vi "Generate command.vi"(1 "Action":T1, 7 "n(0)":i32, 9 "d(0.0)":dbl, 11 "error IO":errorcluster) -> (8 "Command string":string, 10 "Reply expected":bool, 15 "error out":errorcluster)   [LabVIEW 2011]
uses:
  PCP Commands.ctl
  <vilib>/Utility/VariantDataType/VariantType.lvlib
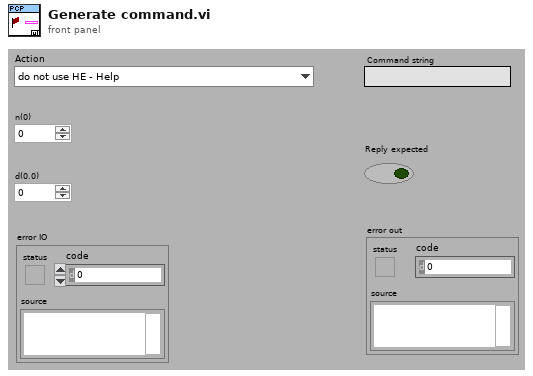
[diagram p1: front panel]
types:
  T1 = typedef "PCP Commands.ctl" = enum16{"do not use HE - Help", "RDd - Most used inputs", "RA - All analog inputs", "RE n Reset DO n", "SE n Set DO n", "RP - Get digital inputs", "VA d Set AO A  Motor Volt", "VB d Set AO B  Cable Resistance", "VEr - Get Version", "DYp - Depth counter", "DR - Reset Depth Counter", "DS n Set Depth options(0-3)", "do not use ME - Manual mode enabled", "MD - Manual mode disabled", "ID - Get ID(2001)", "TS - Get Timestamp", "TO d(s)  Set timeout", "do not use LO n Start Loop Mode(1,2)", "AL n RD&LO variation", "ST - Stop Loop Mode"}
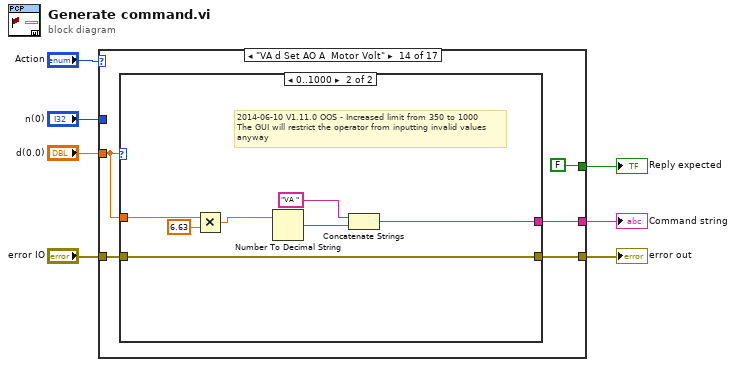
[diagram p0: block diagram]
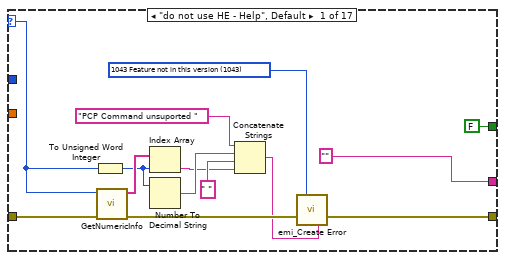
[diagram p2: hidden frame]
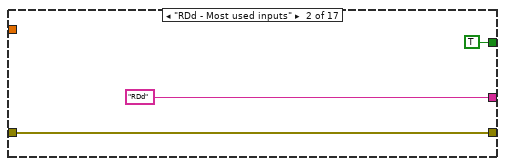
[diagram p3: hidden frame]
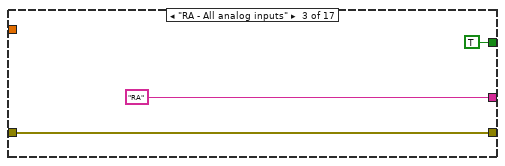
[diagram p4: hidden frame]
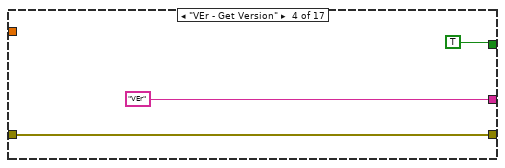
[diagram p5: hidden frame]
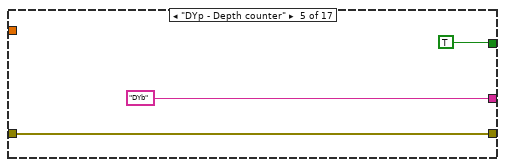
[diagram p6: hidden frame]
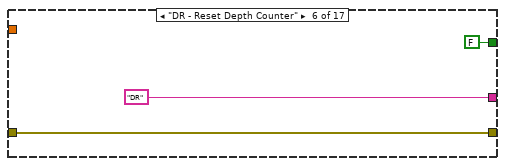
[diagram p7: hidden frame]
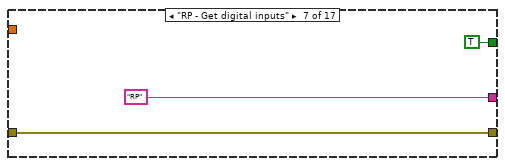
[diagram p8: hidden frame]
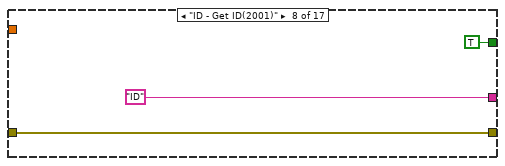
[diagram p9: hidden frame]
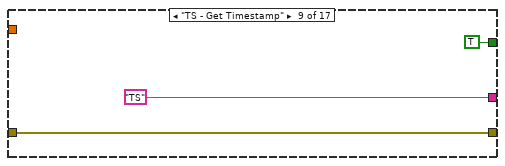
[diagram p10: hidden frame]
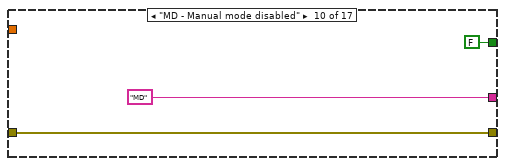
[diagram p11: hidden frame]
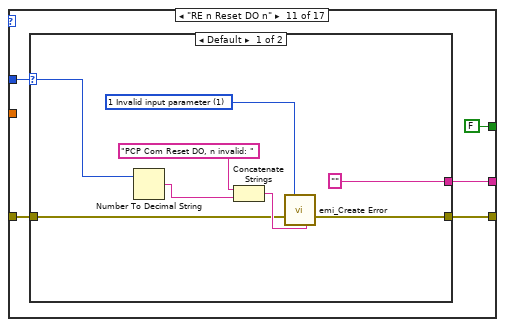
[diagram p12: hidden frame]
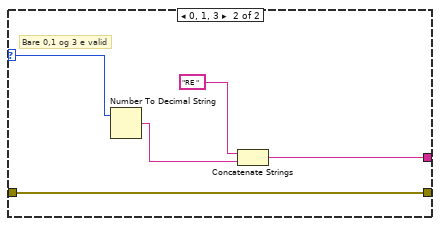
[diagram p13: hidden frame]
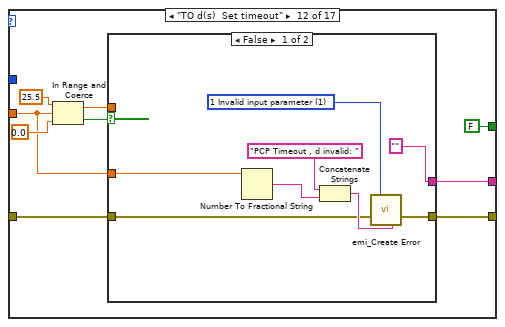
[diagram p14: hidden frame]
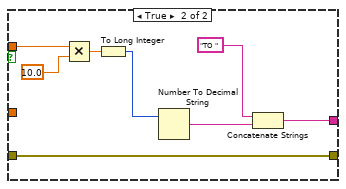
[diagram p15: hidden frame]
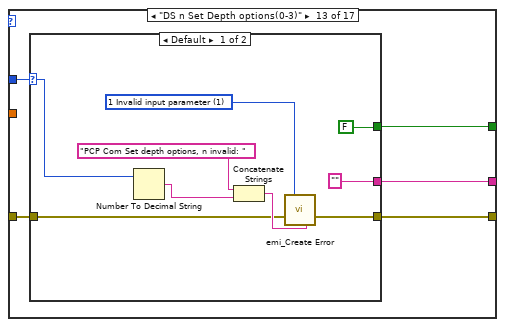
[diagram p16: hidden frame]
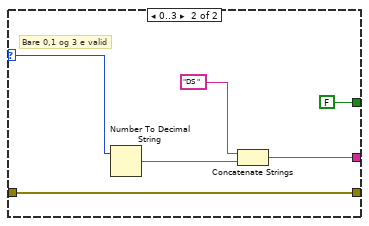
[diagram p17: hidden frame]
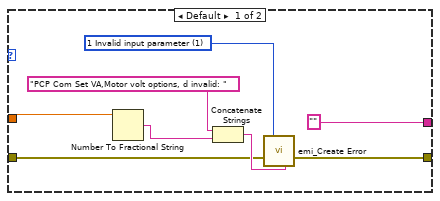
[diagram p18: hidden frame]
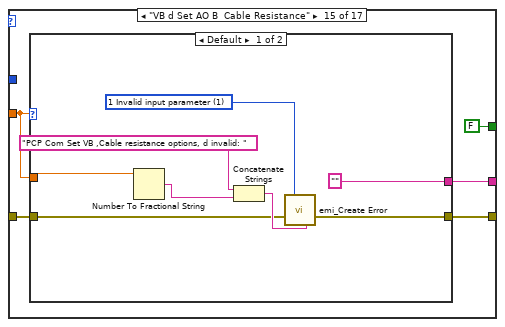
[diagram p19: hidden frame]
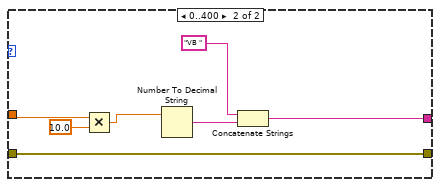
[diagram p20: hidden frame]
diagram:
  n1 = case shown="\"VA d Set AO A  Motor Volt\"" "Action" {
    selector: "Action" -> [w17 _ _ _ _ _ _ _ _ _ _ _ _ _ _ _ _]
    tunnel: "error IO" -> [w19 w24 w27 w30 w33 w36 w39 w42 w45 w48 w51 w74 w94 w115 w135 w154 w172]
    tunnel: [w21 w24 w27 w30 w33 w36 w39 w42 w45 w48 w50 w73 w93 w114 w134 w153 w171] -> w6
    tunnel: "n(0)" -> [_ _ _ _ _ _ _ _ _ _ w52 _ w95 _ _ w155 w173]
    tunnel: ["" "RDd" "RA" "VEr" "DYb" "DR" "RP" "ID" "TS" "MD" w53 w75 w96 w116 w136 w156 w174] -> w7
    tunnel: "d(0.0)" -> [_ _ _ _ _ _ _ _ _ _ _ w67 _ w113 w133 _ _]
    tunnel: [FALSE ("Reply expected") TRUE ("Reply expected") TRUE ("Reply expected") TRUE ("Reply expected") TRUE ("Reply expected") FALSE ("Reply expected") TRUE ("Reply expected") TRUE ("Reply expected") TRUE ("Reply expected") FALSE ("Reply expected") FALSE ("Reply expected") FALSE ("Reply expected") w92 FALSE ("Reply expected") FALSE ("Reply expected") FALSE ("Reply expected") FALSE ("Reply expected")] -> w1
    frame "do not use HE - Help", Default {
      w20 = 1043 items=["0 No Error"=0, "7 File not Found"=7, "35 Generic Pring Error"=35, "37 Device not Found"=37, "39 Device Unit Error"=39, "40 Could fot Open Device"=40, "42 Generic Error"=42, "52 Unknown Message"=52, "98 Bad File type"=98, "99 Bad File Version"=99, "100 Bad Data in File"=100, "1018 Unspecefied Error"=1018, "1041 Incorrect Password"=1041, "1043 Feature not in this version"=1043] ("Error Code")
      n2 = To Unsigned Word Integer(number=w17) -> (unsigned 16bit integer=w15:u16)
      n3 = call <vilib>:"GetNumericInfo.vi"("error in (no error)"=w19, "Variant"=w17) -> ("error out"=w18:errorcluster, "EnumNames"=w16:string[])  [unwired: 6 in, 2 out]
      n4 = Index Array(array=w16, index=w15) -> (element=w11:string)
      n5 = Number To Decimal String(number=w15) -> (decimal integer string=w13:string)  [unwired: 1 in]
      n6 = Concatenate Strings("PCP Command unsuported " ("string"), w13, " " ("string"), w11) -> (w10:string)
      n7 = call "emi_Create Error.vi"("Error Code"=w20, "error in (no error)"=w18, "Append String(\"\")"=w10) -> ("error out"=w21:errorcluster)  [unwired: 12 in]
    }
    frame "RDd - Most used inputs" {
    }
    frame "RA - All analog inputs" {
    }
    frame "VEr - Get Version" {
    }
    frame "DYp - Depth counter" {
    }
    frame "DR - Reset Depth Counter" {
    }
    frame "RP - Get digital inputs" {
    }
    frame "ID - Get ID(2001)" {
    }
    frame "TS - Get Timestamp" {
    }
    frame "MD - Manual mode disabled" {
    }
    frame "RE n Reset DO n" {
      n8 = case shown="Default" w52 {
        selector: w52 -> [w56 w64]
        tunnel: ["" w65] -> w53
        tunnel: w51 -> [w54 w62]
        tunnel: [w55 w62] -> w50
        frame Default {
          w60 = 1 items=["0 No Error"=0, "1 Invalid input parameter"=1, "6 Generic file IO "=6, "7 File not Found"=7, "35 Generic Pring Error"=35, "37 Device not Found"=37, "39 Device Unit Error"=39, "40 Could fot Open Device"=40, "42 Generic Error"=42, "52 Unknown Message"=52, "98 Bad File type"=98, "99 Bad File Version"=99, "100 Bad Data in File"=100, "1018 Unspecefied Error"=1018, "1041 Incorrect Password"=1041, "1043 Feature not in this version"=1043] ("Error Code")
          n9 = Number To Decimal String(number=w56) -> (decimal integer string=w57:string)  [unwired: 1 in]
          n10 = Concatenate Strings("PCP Com Reset DO, n invalid: " ("string"), w57) -> (w59:string)
          n11 = call "emi_Create Error.vi"("Error Code"=w60, "error in (no error)"=w54, "Append String(\"\")"=w59) -> ("error out"=w55:errorcluster)  [unwired: 12 in]
        }
        frame 0, 1, 3 {
          # "Bare 0,1 og 3 e valid"
          n12 = Number To Decimal String(number=w64) -> (decimal integer string=w63:string)  [unwired: 1 in]
          n13 = Concatenate Strings("RE ", w63) -> (w65:string)
        }
      }
    }
    frame "TO d(s)  Set timeout" {
      n14 = In Range and Coerce(upper limit=25.5, x=w67, lower limit=0.0) -> (coerced(x)=w69:dbl, In Range?=w68:bool)
      n15 = case shown="False" w68 {
        tunnel: ["" w90] -> w75
        tunnel: w74 -> [w76 w89]
        tunnel: [w77 w89] -> w73
        tunnel: w69 -> [_ w88]
        tunnel: w67 -> [w78 _]
        frame False {
          w82 = 1 items=["0 No Error"=0, "1 Invalid input parameter"=1, "6 Generic file IO "=6, "7 File not Found"=7, "35 Generic Pring Error"=35, "37 Device not Found"=37, "39 Device Unit Error"=39, "40 Could fot Open Device"=40, "42 Generic Error"=42, "52 Unknown Message"=52, "98 Bad File type"=98, "99 Bad File Version"=99, "100 Bad Data in File"=100, "1018 Unspecefied Error"=1018, "1041 Incorrect Password"=1041, "1043 Feature not in this version"=1043] ("Error Code")
          n16 = Number To Fractional String(number=w78) -> (F-format string=w79:string)  [unwired: 3 in]
          n17 = Concatenate Strings("PCP Timeout , d invalid: " ("string"), w79) -> (w81:string)
          n18 = call "emi_Create Error.vi"("Error Code"=w82, "error in (no error)"=w76, "Append String(\"\")"=w81) -> ("error out"=w77:errorcluster)  [unwired: 12 in]
        }
        frame True {
          n19 = Multiply(x=w88, y=10.0) -> (x*y=w85:dbl)
          n20 = To Long Integer(number=w85) -> (32bit integer=w84:i32)
          n21 = Number To Decimal String(number=w84) -> (decimal integer string=w86:string)  [unwired: 1 in]
          n22 = Concatenate Strings("TO ", w86) -> (w90:string)
        }
      }
    }
    frame "DS n Set Depth options(0-3)" {
      n23 = case shown="Default" w95 {
        selector: w95 -> [w100 w109]
        tunnel: ["" w110] -> w96
        tunnel: w94 -> [w97 w107]
        tunnel: [w98 w107] -> w93
        tunnel: [FALSE ("Reply expected") FALSE ("Reply expected")] -> w92
        frame Default {
          w104 = 1 items=["0 No Error"=0, "1 Invalid input parameter"=1, "6 Generic file IO "=6, "7 File not Found"=7, "35 Generic Pring Error"=35, "37 Device not Found"=37, "39 Device Unit Error"=39, "40 Could fot Open Device"=40, "42 Generic Error"=42, "52 Unknown Message"=52, "98 Bad File type"=98, "99 Bad File Version"=99, "100 Bad Data in File"=100, "1018 Unspecefied Error"=1018, "1041 Incorrect Password"=1041, "1043 Feature not in this version"=1043] ("Error Code")
          n24 = Number To Decimal String(number=w100) -> (decimal integer string=w101:string)  [unwired: 1 in]
          n25 = Concatenate Strings("PCP Com Set depth options, n invalid: " ("string"), w101) -> (w103:string)
          n26 = call "emi_Create Error.vi"("Error Code"=w104, "error in (no error)"=w97, "Append String(\"\")"=w103) -> ("error out"=w98:errorcluster)  [unwired: 12 in]
        }
        frame 0..3 {
          # "Bare 0,1 og 3 e valid"
          n27 = Number To Decimal String(number=w109) -> (decimal integer string=w108:string)  [unwired: 1 in]
          n28 = Concatenate Strings("DS ", w108) -> (w110:string)
        }
      }
    }
    frame "VA d Set AO A  Motor Volt" {
      n29 = case shown="0..1000" w113 {
        tunnel: ["" w130] -> w116
        tunnel: w115 -> [w117 w128]
        tunnel: [w118 w128] -> w114
        tunnel: w113 -> [w119 w127]
        frame Default {
          w123 = 1 items=["0 No Error"=0, "1 Invalid input parameter"=1, "6 Generic file IO "=6, "7 File not Found"=7, "35 Generic Pring Error"=35, "37 Device not Found"=37, "39 Device Unit Error"=39, "40 Could fot Open Device"=40, "42 Generic Error"=42, "52 Unknown Message"=52, "98 Bad File type"=98, "99 Bad File Version"=99, "100 Bad Data in File"=100, "1018 Unspecefied Error"=1018, "1041 Incorrect Password"=1041, "1043 Feature not in this version"=1043] ("Error Code")
          n30 = Number To Fractional String(number=w119) -> (F-format string=w120:string)  [unwired: 3 in]
          n31 = Concatenate Strings("PCP Com Set VA,Motor volt options, d invalid: " ("string"), w120) -> (w122:string)
          n32 = call "emi_Create Error.vi"("Error Code"=w123, "error in (no error)"=w117, "Append String(\"\")"=w122) -> ("error out"=w118:errorcluster)  [unwired: 12 in]
        }
        frame 0..1000 {
          # "2014-06-10 V1.11.0 OOS - Increased limit from 350 to 1000\nThe GUI will restrict the operator from inputting invalid values\nanyway"
          n33 = Multiply(x=w127, y=6.63) -> (x*y=w125:dbl)
          n34 = Number To Decimal String(number=w125) -> (decimal integer string=w129:string)  [unwired: 1 in]
          n35 = Concatenate Strings("VA ", w129) -> (w130:string)
        }
      }
    }
    frame "VB d Set AO B  Cable Resistance" {
      n36 = case shown="Default" w133 {
        tunnel: ["" w150] -> w136
        tunnel: w135 -> [w138 w148]
        tunnel: [w137 w148] -> w134
        tunnel: w133 -> [w139 w147]
        frame Default {
          w143 = 1 items=["0 No Error"=0, "1 Invalid input parameter"=1, "6 Generic file IO "=6, "7 File not Found"=7, "35 Generic Pring Error"=35, "37 Device not Found"=37, "39 Device Unit Error"=39, "40 Could fot Open Device"=40, "42 Generic Error"=42, "52 Unknown Message"=52, "98 Bad File type"=98, "99 Bad File Version"=99, "100 Bad Data in File"=100, "1018 Unspecefied Error"=1018, "1041 Incorrect Password"=1041, "1043 Feature not in this version"=1043] ("Error Code")
          n37 = Number To Fractional String(number=w139) -> (F-format string=w140:string)  [unwired: 3 in]
          n38 = Concatenate Strings("PCP Com Set VB ,Cable resistance options, d invalid: " ("string"), w140) -> (w142:string)
          n39 = call "emi_Create Error.vi"("Error Code"=w143, "error in (no error)"=w138, "Append String(\"\")"=w142) -> ("error out"=w137:errorcluster)  [unwired: 12 in]
        }
        frame 0..400 {
          n40 = Multiply(x=w147, y=10.0) -> (x*y=w145:dbl)
          n41 = Number To Decimal String(number=w145) -> (decimal integer string=w149:string)  [unwired: 1 in]
          n42 = Concatenate Strings("VB ", w149) -> (w150:string)
        }
      }
    }
    frame "SE n Set DO n" {
      n43 = case shown="0, 1, 3" w155 {
        selector: w155 -> [w159 w167]
        tunnel: ["" w168] -> w156
        tunnel: w154 -> [w157 w165]
        tunnel: [w158 w165] -> w153
        frame Default {
          w163 = 1 items=["0 No Error"=0, "1 Invalid input parameter"=1, "6 Generic file IO "=6, "7 File not Found"=7, "35 Generic Pring Error"=35, "37 Device not Found"=37, "39 Device Unit Error"=39, "40 Could fot Open Device"=40, "42 Generic Error"=42, "52 Unknown Message"=52, "98 Bad File type"=98, "99 Bad File Version"=99, "100 Bad Data in File"=100, "1018 Unspecefied Error"=1018, "1041 Incorrect Password"=1041, "1043 Feature not in this version"=1043] ("Error Code")
          n44 = Number To Decimal String(number=w159) -> (decimal integer string=w160:string)  [unwired: 1 in]
          n45 = Concatenate Strings("PCP Com Set DO, n invalid: " ("string"), w160) -> (w162:string)
          n46 = call "emi_Create Error.vi"("Error Code"=w163, "error in (no error)"=w157, "Append String(\"\")"=w162) -> ("error out"=w158:errorcluster)  [unwired: 12 in]
        }
        frame 0, 1, 3 {
          # "Bare 0,1 og 3 e valid"
          n47 = Number To Decimal String(number=w167) -> (decimal integer string=w166:string)  [unwired: 1 in]
          n48 = Concatenate Strings("SE ", w166) -> (w168:string)
        }
      }
    }
    frame "AL n RD&LO variation" {
      n49 = case shown="Default" w173 {
        selector: w173 -> [w177 w185]
        tunnel: ["" w186] -> w174
        tunnel: w172 -> [w175 w183]
        tunnel: [w176 w183] -> w171
        frame Default {
          w181 = 1 items=["0 No Error"=0, "1 Invalid input parameter"=1, "6 Generic file IO "=6, "7 File not Found"=7, "35 Generic Pring Error"=35, "37 Device not Found"=37, "39 Device Unit Error"=39, "40 Could fot Open Device"=40, "42 Generic Error"=42, "52 Unknown Message"=52, "98 Bad File type"=98, "99 Bad File Version"=99, "100 Bad Data in File"=100, "1018 Unspecefied Error"=1018, "1041 Incorrect Password"=1041, "1043 Feature not in this version"=1043] ("Error Code")
          n50 = Number To Decimal String(number=w177) -> (decimal integer string=w178:string)  [unwired: 1 in]
          n51 = Concatenate Strings("PCP AL, com variation, n invalid: " ("string"), w178) -> (w180:string)
          n52 = call "emi_Create Error.vi"("Error Code"=w181, "error in (no error)"=w175, "Append String(\"\")"=w180) -> ("error out"=w176:errorcluster)  [unwired: 12 in]
        }
        frame 0, 1 {
          # "Bare 0,1 e valid"
          n53 = Number To Decimal String(number=w185) -> (decimal integer string=w184:string)  [unwired: 1 in]
          n54 = Concatenate Strings("AL ", w184) -> (w186:string)
        }
      }
    }
  }
  "Command string" <- w7
  "error out" <- w6
  "Reply expected" <- w1
